vi "stabilizePress_05.vi"() -> ()   [LabVIEW 2011]
panel:
  out "tElaps":dbl=32.29700000002049
  in  "dT_fit(s)":dbl=1.0
  in  "tTotal(s)":dbl=30.0
  out "tNow":dbl=343296.145
  out "XY Graph":cluster{"Value":dbl[], "Value":dbl[]}(graph)={"Value"=[1.5420000000158325, 3.0790000000270084, 4.619000000006054, 6.157000000006519, 7.695000000006985, 9.23300000000745, 10.772999999986496, 12.309999999997672, 13.847000000008848, 15.386999999987893, 16.92399999999907, 18.462999999988824, 19.99900000001071, 21.53499999997439, 23.07400000002235, 24.61099999997532, 26.147999999986496, 27.68499999999767, 29.222999999998137, 30.760999999998603, 32.29700000002049], "Value"=[16.36, 19.38, 18.91, 17.669999999999998, 16.93, 17.98, 18.610000000000003, 18.83, 19.259999999999998, 19.459999999999997, 19.55, 19.71, 19.91, 19.939999999999998, 19.92, 19.939999999999998, 19.959999999999997, 19.959999999999997, 19.950000000000003, 19.950000000000003, 20.01]}
  out "tune Setpoint(torr)":dbl=20.0
  in  "t array":dbl[](array[numeric])=[1.5420000000158325, 3.0790000000270084, 4.619000000006054, 6.157000000006519, 7.695000000006985, 9.23300000000745, 10.772999999986496, 12.309999999997672, 13.847000000008848, 15.386999999987893, 16.92399999999907, 18.462999999988824, 19.99900000001071, 21.53499999997439, 23.07400000002235, 24.61099999997532, 26.147999999986496, 27.68499999999767, 29.222999999998137, 30.760999999998603, 32.29700000002049]
  out "P array":dbl[](array[numeric])=[16.36, 19.38, 18.91, 17.669999999999998, 16.93, 17.98, 18.610000000000003, 18.83, 19.259999999999998, 19.459999999999997, 19.55, 19.71, 19.91, 19.939999999999998, 19.92, 19.939999999999998, 19.959999999999997, 19.959999999999997, 19.950000000000003, 19.950000000000003, 20.01]
  out "stabilize done":bool=TRUE
  in  "tExp(s)":dbl=15.0
  out "Set Point (torr)":dbl=20.0 format="%.2f"
  out "Setpoint Index":string="C"
  out "Setpoint Index control":u16(ring)=2 caption="Setpoint" items=["A", "B", "C", "D"]
  out "first":bool
  out "tStart":dbl=343263.848
  in  "time done (s)":dbl
  out "Wait to set":bool
  out "IO error":errorcluster={"status"=FALSE, "code"=1073676418, "source"="VISA Close in WriteAdaptorr04.vi->writeSetPoint_01.vi->stabilizePress_05.vi"}
  in  "stop":bool
  out "P (torr)":dbl=20.01 format="%.2f"
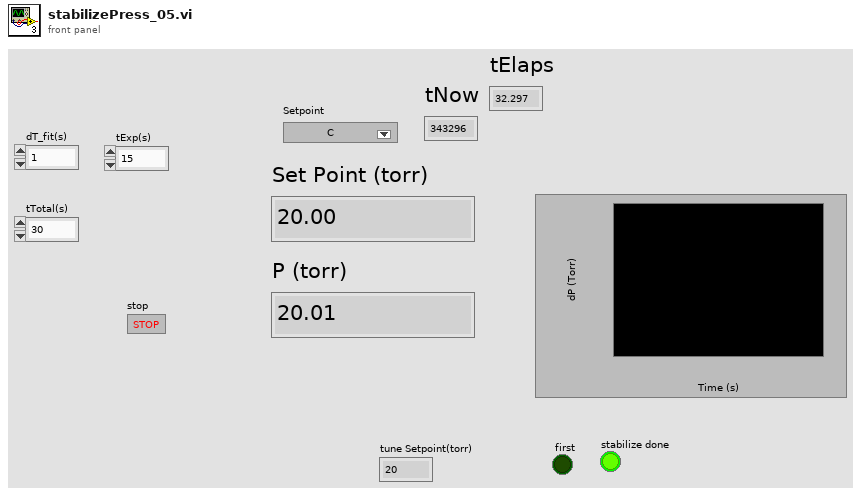
[diagram p1: front panel]
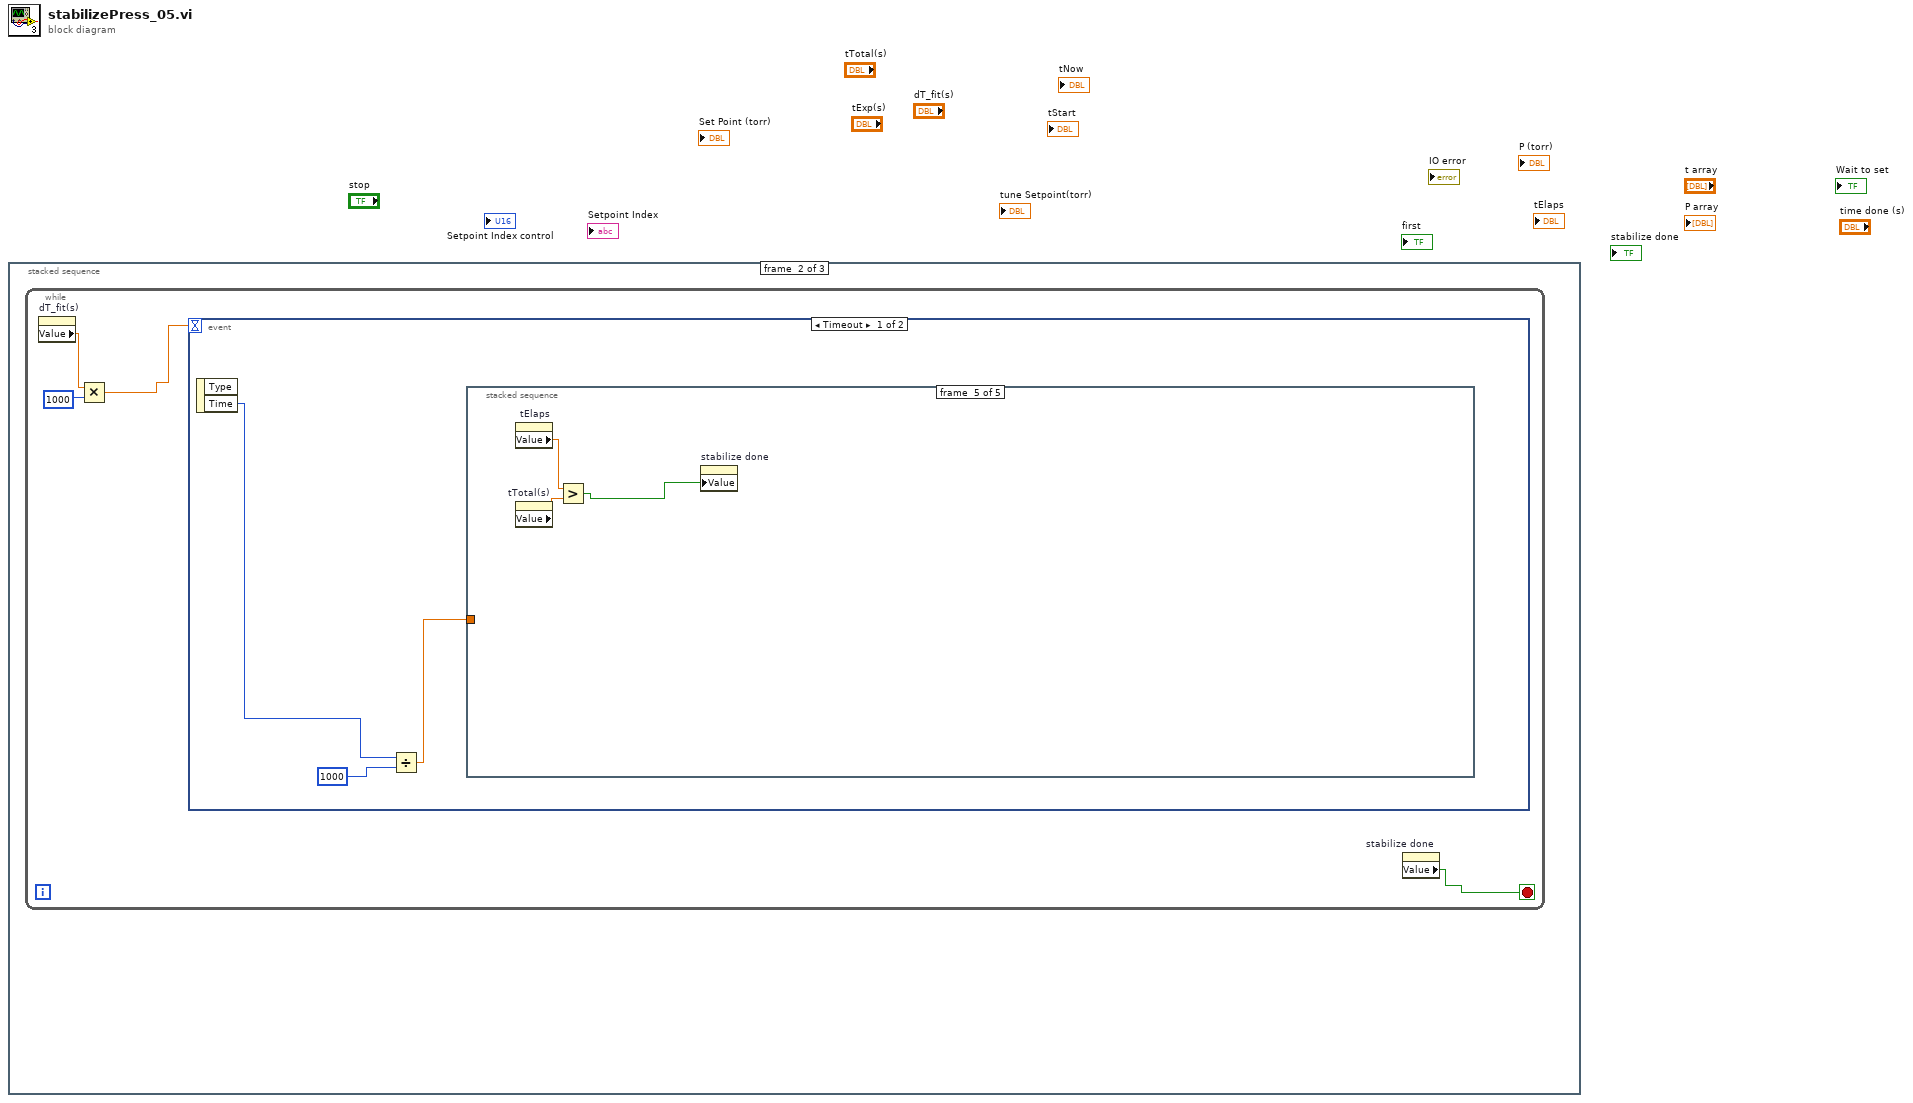
[diagram p0: block diagram]
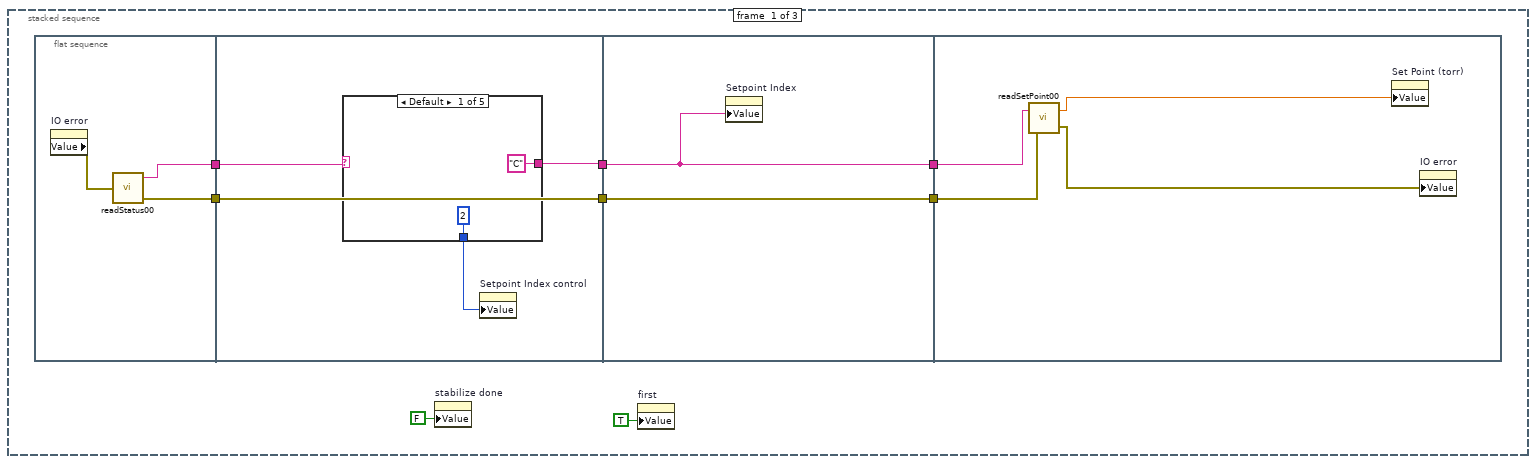
[diagram p2: hidden frame]
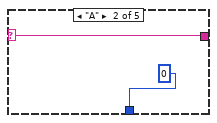
[diagram p3: hidden frame]
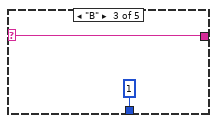
[diagram p4: hidden frame]
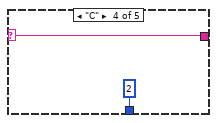
[diagram p5: hidden frame]
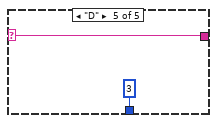
[diagram p6: hidden frame]
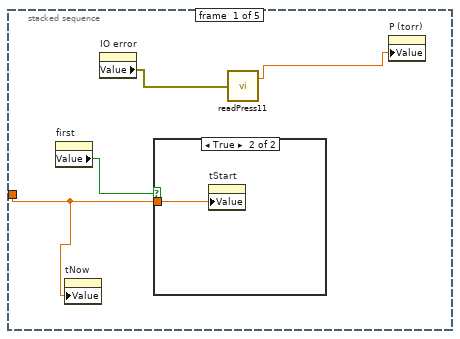
[diagram p7: hidden frame]
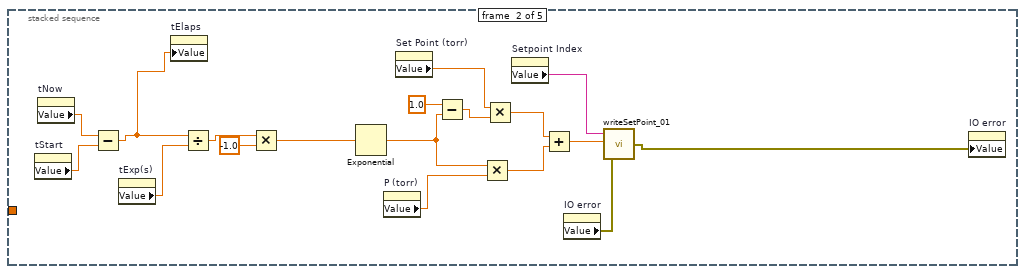
[diagram p9: hidden frame]
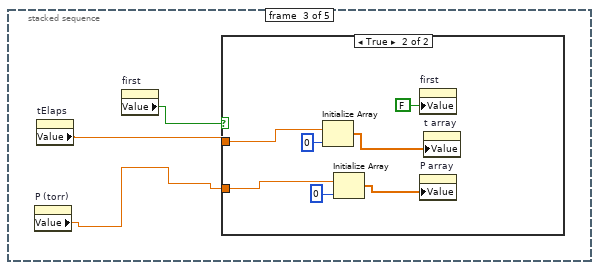
[diagram p10: hidden frame]
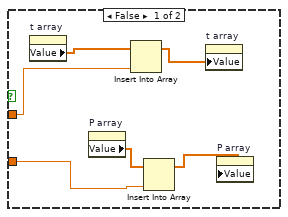
[diagram p11: hidden frame]
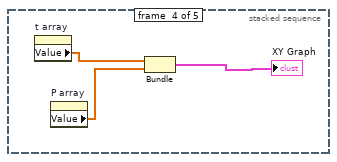
[diagram p12: hidden frame]
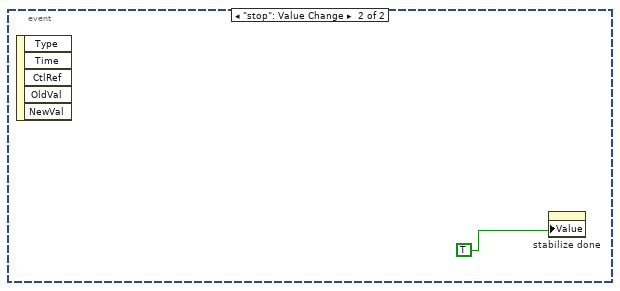
[diagram p13: hidden frame]
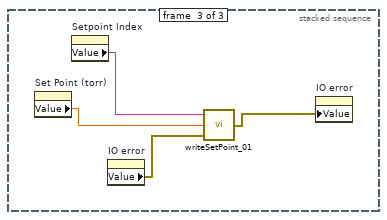
[diagram p14: hidden frame]
diagram:
  n1 = stacked-sequence {
    frame #0 {
      n2 = flat-sequence {
        tunnel: [w10] -> w8
        tunnel: [w9] -> w7
        tunnel: w8 -> [w14]
        tunnel: [w13] -> w6
        tunnel: w7 -> [w15]
        tunnel: [w15] -> w5
        tunnel: w6 -> [w26]
        tunnel: [w26] -> w4
        tunnel: w5 -> [w27]
        tunnel: [w27] -> w3
        tunnel: w4 -> [w31]
        tunnel: w3 -> [w30]
        frame #0 {
          n3 = property on="IO error" class="Clust (strict)"() -> ("Value"=w11:errorcluster)  [unwired: 2 in, 2 out]
          n4 = call "readStatus00.vi"("error in"=w11) -> ("Setpoint"=w10:string, "error out"=w9:errorcluster)  [unwired: 1 out]
        }
        frame #1 {
          n5 = case shown="Default" w14 {
            selector: w14 -> [_ w19 w20 w22 w24]
            tunnel: ["C" w19 w20 w22 w24] -> w13
            tunnel: [u16 2 ("Ring") u16 0 ("Ring") u16 1 ("Ring") u16 2 ("Ring") u16 3 ("Ring")] -> w12
            frame Default {
            }
            frame "A" {
            }
            frame "B" {
            }
            frame "C" {
            }
            frame "D" {
            }
          }
          n6 = property on="Setpoint Index control" class="Ring (strict)"("Value"=w12) -> ()  [unwired: 2 in, 2 out]
        }
        frame #2 {
          n7 = property on="Setpoint Index" class="Str"("Value"=w26) -> ()  [unwired: 2 in, 2 out]
        }
        frame #3 {
          n8 = call "readSetPoint00.vi"("error in"=w30, "Setpoint"=w31) -> ("error out"=w29:errorcluster, "P"=w28:dbl)
          n9 = property on="Set Point (torr)" class="DigNum (strict)"("Value"=w28) -> ()  [unwired: 2 in, 2 out]
          n10 = property on="IO error" class="Clust (strict)"("Value"=w29) -> ()  [unwired: 2 in, 2 out]
        }
      }
      n11 = property on="stabilize done" class="Bool (strict)"("Value"=FALSE ("fit done")) -> ()  [unwired: 2 in, 2 out]
      n12 = property on="first" class="Bool (strict)"("Value"=TRUE ("first")) -> ()  [unwired: 2 in, 2 out]
    }
    frame #1 {
      n13 = while {
        stop <- w32 stop-if-true
        n14 = property on="dT_fit(s)" class="DigNum (strict)"() -> ("Value"=w34:dbl)  [unwired: 2 in, 2 out]
        n15 = Multiply(x=w34, y=u32 1000) -> (x*y=w33:dbl)
        n16 = event shown="[0] Timeout" {
          selector: _ -> [_ _]
          dyn-events: _ -> [_ _]
          timeout: w33 -> [_ _]
          event Timeout {
            n17 = event-data() -> ("Time"=w36:u32)  [unwired: 1 in, 1 out]
            n18 = Divide(x=w36, y=i64 1000) -> (x/y=w37:dbl)
            n19 = stacked-sequence {
              tunnel: w37 -> [w39 _ _ _ _]
              frame #0 {
                n20 = property on="first" class="Bool (strict)"() -> ("Value"=w41:bool)  [unwired: 2 in, 2 out]
                n21 = property on="tNow" class="DigNum (strict)"("Value"=w39) -> ()  [unwired: 2 in, 2 out]
                n22 = property on="IO error" class="Clust (strict)"() -> ("Value"=w42:errorcluster)  [unwired: 2 in, 2 out]
                n23 = case shown="True" w41 {
                  tunnel: w39 -> [_ w43]
                  frame False {
                  }
                  frame True {
                    n24 = property on="tStart" class="DigNum (strict)"("Value"=w43) -> ()  [unwired: 2 in, 2 out]
                  }
                }
                n25 = call "readPress11.vi"("error in"=w42) -> ("P"=w40:dbl)  [unwired: 1 out]
                n26 = property on="P (torr)" class="DigNum (strict)"("Value"=w40) -> ()  [unwired: 2 in, 2 out]
              }
              frame #1 {
                n27 = property on="tStart" class="DigNum (strict)"() -> ("Value"=w60:dbl)  [unwired: 2 in, 2 out]
                n28 = property on="tNow" class="DigNum (strict)"() -> ("Value"=w61:dbl)  [unwired: 2 in, 2 out]
                n29 = Subtract(x=w61, y=w60) -> (x-y=w44:dbl)
                n30 = property on="tExp(s)" class="DigNum (strict)"() -> ("Value"=w59:dbl)  [unwired: 2 in, 2 out]
                n31 = property on="tElaps" class="DigNum (strict)"("Value"=w44) -> ()  [unwired: 2 in, 2 out]
                n32 = Divide(x=w44, y=w59) -> (x/y=w58:dbl)
                n33 = Multiply(x=w58, y=-1.0) -> (x*y=w56:dbl)
                n34 = Exponential(1:w56) -> (0:w51:dbl)
                n35 = property on="P (torr)" class="DigNum (strict)"() -> ("Value"=w52:dbl)  [unwired: 2 in, 2 out]
                n36 = property on="Set Point (torr)" class="DigNum (strict)"() -> ("Value"=w53:dbl)  [unwired: 2 in, 2 out]
                n37 = Subtract(x=1.0, y=w51) -> (x-y=w54:dbl)
                n38 = Multiply(x=w51, y=w52) -> (x*y=w49:dbl)
                n39 = Multiply(x=w53, y=w54) -> (x*y=w50:dbl)
                n40 = property on="Setpoint Index" class="Str"() -> ("Value"=w47:string)  [unwired: 2 in, 2 out]
                n41 = Add(x=w50, y=w49) -> (x+y=w48:dbl)
                n42 = property on="IO error" class="Clust (strict)"() -> ("Value"=w46:errorcluster)  [unwired: 2 in, 2 out]
                n43 = call "writeSetPoint_01.vi"("error in"=w46, "P (Torr)"=w48, "Setpoint"=w47) -> ("error out"=w45:errorcluster)
                n44 = property on="IO error" class="Clust (strict)"("Value"=w45) -> ()  [unwired: 2 in, 2 out]
              }
              frame #2 {
                n45 = property on="P (torr)" class="DigNum (strict)"() -> ("Value"=w63:dbl)  [unwired: 2 in, 2 out]
                n46 = property on="tElaps" class="DigNum (strict)"() -> ("Value"=w62:dbl)  [unwired: 2 in, 2 out]
                n47 = property on="first" class="Bool (strict)"() -> ("Value"=w64:bool)  [unwired: 2 in, 2 out]
                n48 = case shown="True" w64 {
                  tunnel: w63 -> [w70 w76]
                  tunnel: w62 -> [w67 w74]
                  frame False {
                    n49 = property on="t array" class="Arr (strict)"() -> ("Value"=w66:dbl[])  [unwired: 2 in, 2 out]
                    n50 = property on="P array" class="Arr (strict)"() -> ("Value"=w68:dbl[])  [unwired: 2 in, 2 out]
                    n51 = Insert Into Array(array=w66, new element=w67) -> (w65:dbl[])  [unwired: 1 in]
                    n52 = Insert Into Array(array=w68, new element=w70) -> (w69:dbl[])  [unwired: 1 in]
                    n53 = property on="t array" class="Arr (strict)"("Value"=w65) -> ()  [unwired: 2 in, 2 out]
                    n54 = property on="P array" class="Arr (strict)"("Value"=w69) -> ()  [unwired: 2 in, 2 out]
                  }
                  frame True {
                    n55 = Initialize Array(w74, 0 ("dimension size")) -> (w71:dbl[])
                    n56 = Initialize Array(w76, 0 ("dimension size")) -> (w72:dbl[])
                    n57 = property on="first" class="Bool (strict)"("Value"=FALSE ("first")) -> ()  [unwired: 2 in, 2 out]
                    n58 = property on="P array" class="Arr (strict)"("Value"=w72) -> ()  [unwired: 2 in, 2 out]
                    n59 = property on="t array" class="Arr (strict)"("Value"=w71) -> ()  [unwired: 2 in, 2 out]
                  }
                }
              }
              frame #3 {
                n60 = property on="t array" class="Arr (strict)"() -> ("Value"=w79:dbl[])  [unwired: 2 in, 2 out]
                n61 = property on="P array" class="Arr (strict)"() -> ("Value"=w80:dbl[])  [unwired: 2 in, 2 out]
                n62 = Bundle "Bundle"("Value"=w79, "Value"=w80) -> (→"XY Graph":cluster{"Value":dbl[], "Value":dbl[]})  [unwired: 1 in]
              }
              frame #4 {
                n63 = property on="tElaps" class="DigNum (strict)"() -> ("Value"=w82:dbl)  [unwired: 2 in, 2 out]
                n64 = property on="tTotal(s)" class="DigNum (strict)"() -> ("Value"=w83:dbl)  [unwired: 2 in, 2 out]
                n65 = Greater?(x=w82, y=w83) -> (0:w81:bool)
                n66 = property on="stabilize done" class="Bool (strict)"("Value"=w81) -> ()  [unwired: 2 in, 2 out]
              }
            }
          }
          event "stop": Value Change {
            n67 = event-data() -> ()  [unwired: 1 in, 5 out]
            n68 = property on="stabilize done" class="Bool (strict)"("Value"=TRUE ("stabilize done")) -> ()  [unwired: 2 in, 2 out]
          }
        }
        n69 = property on="stabilize done" class="Bool (strict)"() -> ("Value"=w32:bool)  [unwired: 2 in, 2 out]
      }
    }
    frame #2 {
      n70 = property on="Set Point (torr)" class="DigNum (strict)"() -> ("Value"=w88:dbl)  [unwired: 2 in, 2 out]
      n71 = property on="Setpoint Index" class="Str"() -> ("Value"=w87:string)  [unwired: 2 in, 2 out]
      n72 = property on="IO error" class="Clust (strict)"() -> ("Value"=w86:errorcluster)  [unwired: 2 in, 2 out]
      n73 = call "writeSetPoint_01.vi"("error in"=w86, "P (Torr)"=w88, "Setpoint"=w87) -> ("error out"=w85:errorcluster)
      n74 = property on="IO error" class="Clust (strict)"("Value"=w85) -> ()  [unwired: 2 in, 2 out]
    }
  }
